vi "FTW-Endpoint-Connect.vi"(0 "FTW Endpoint":refnum<class "FTW-Endpoint-TCP.lvclass">, 5 "Endpoint Address":string, 11 "error in":errorcluster) -> (4 "FTW Endpoint out":refnum<class "FTW-Endpoint-TCP.lvclass">, 15 "error out":errorcluster)   [LabVIEW 2013, in "FTW-Endpoint-TCP.lvclass"]
uses:
  FTW-Endpoint-TCP.lvclass
  FTW-Endpoint-TCP.lvclass/FTW-Endpoint-TCP.ctl
panel:
  # "Inputs"
  # "Outputs"
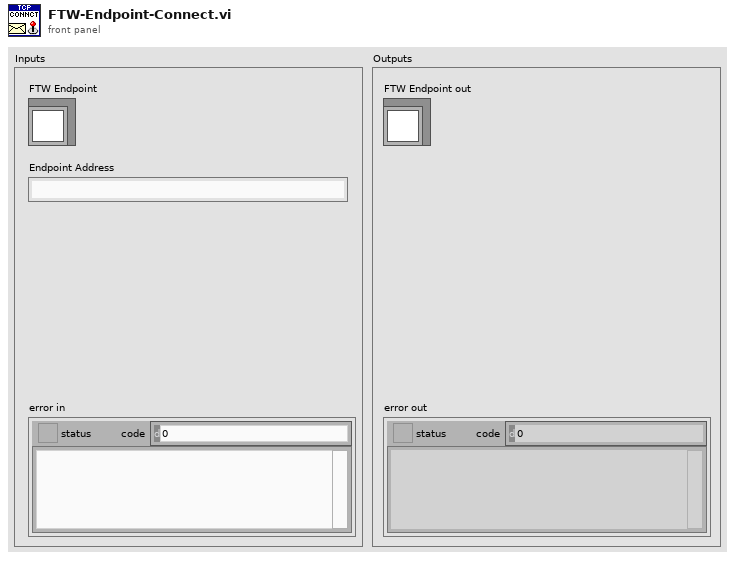
[diagram p1: front panel]
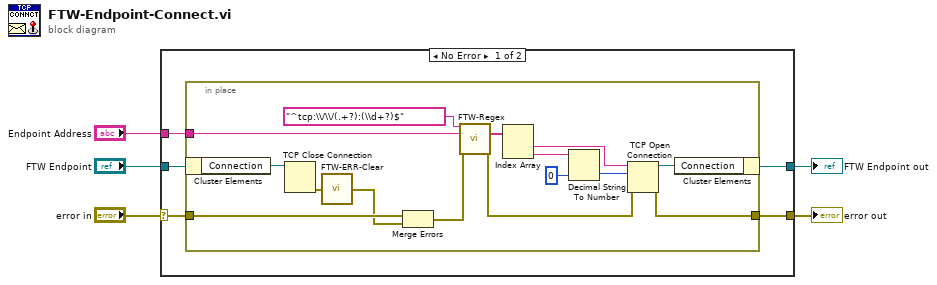
[diagram p0: block diagram]
diagram:
  n1 = case shown="No Error" "error in" {
    selector: "error in" -> [w9 w27]
    tunnel: [w6 w27] -> w5
    tunnel: [w7 w26] -> w3
    tunnel: "FTW Endpoint" -> [w10 w26]
    tunnel: "Endpoint Address" -> [w8 _]
    frame No Error {
      n2 = in-place {
        in-place-border: w9 -> [w16]
        in-place-border: [w18] -> w6
        in-place-border: w8 -> [w14]
        n3 = in-place-cluster #1(w10) -> ("Connection"=w25:refnum<k5>)
        n4 = TCP Close Connection(connection ID=w25) -> (error out=w21:errorcluster)  [unwired: 2 in, 1 out]
        n5 = call "FTW-ERR-Clear.vi"("error to snuff"=w21) -> ("no error"=w12:errorcluster)
        n6 = Merge Errors(w16, w12) -> (w13:errorcluster)
        n7 = call "FTW-Regex.vi"("Regular Expression"="^tcp:\\/\\/(.+?):(\\d+?)$" ("input string"), "Input String"=w14, "error in"=w13) -> ("Submatches"=w24:string[], "error out"=w15:errorcluster)  [unwired: 8 in, 3 out]
        n8 = Index Array(array=w24) -> (element #1=w11:string, element #2=w23:string)  [unwired: 2 in]
        n9 = Decimal String To Number(string=w23, default (0L)=u16 0 ("remote port or service name")) -> (number=w17:u16)  [unwired: 1 in, 1 out]
        n10 = TCP Open Connection(address=w11, remote port or service name=w17, error in (no error)=w15) -> (connection ID=w19:refnum<k5>, error out=w18:errorcluster)  [unwired: 2 in]
        n11 = in-place-cluster #1("Connection"=w19) -> (w7:refnum<class "FTW-Endpoint-TCP.lvclass">)
      }
    }
    frame Error {
    }
  }
  "error out" <- w5
  "FTW Endpoint out" <- w3
